vi "Update Time.vi"(8 "error in":errorcluster) -> (0 "error out":errorcluster)   [LabVIEW 2015]
uses:
  <vilib>/nisyscfg/nisyscfg.lvlib
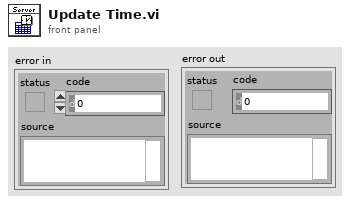
[diagram p1: front panel]
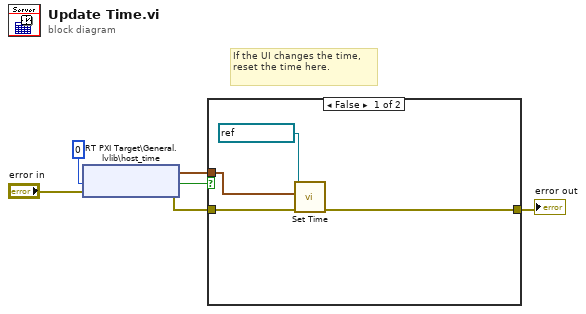
[diagram p0: block diagram]
diagram:
  # "If the UI changes the time, reset the time here."
  n1 = shared-variable "RT PXI Target\\General.lvlib\\host_time"(error in="error in", 0 ("ms timeout (0)")) -> (w4:timestamp, error out=w3:errorcluster, w2:bool)
  n2 = case shown="False" w2 {
    tunnel: w3 -> [w9 w11]
    tunnel: w4 -> [w10 _]
    tunnel: [w8 w11] -> w5
    frame False {
      n3 = call <vilib>:"Set Time.vi"("error in (no error)"=w9, "Time"=w10, "Session in (localhost)"=refnum<k21> "localhost" ("session in (localhost)")) -> ("error out"=w8:errorcluster)  [unwired: 5 in, 3 out]
    }
    frame True {
    }
  }
  "error out" <- w5
